vi "Data.vi"(11 "Helper Loop Create Msg in":refnum<class "Helper Loop Create Msg.lvclass">) -> (2 "Helper Loop":refnum<class "Helper Loop.lvclass">)   [LabVIEW 2021, in "Helper Loop Create.lvlib" / "Helper Loop Create Msg.lvclass"]
uses:
  Helper Loop Create Msg.lvclass
  Helper Loop/Helper Loop.lvclass
  Helper Loop Create Msg.lvclass/Helper Loop Create Msg.ctl
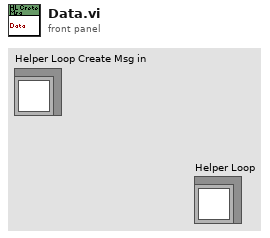
[diagram p1: front panel]
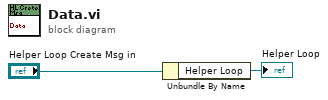
[diagram p0: block diagram]
diagram:
  n1 = Unbundle By Name("Helper Loop Create Msg in") -> ("Helper Loop"=→"Helper Loop":refnum<class "Helper Loop.lvclass">)
